vi "testTTL_v5.vi"() -> ()   [LabVIEW 2015]
uses:
  <vilib>/DAQmx/read.llb/DAQmx Read (Counter U32 1Chan 1Samp).vi
  <vilib>/DAQmx/write.llb/DAQmx Write (Analog Wfm 1Chan NSamp).vi
  <vilib>/DAQmx/write.llb/DAQmx Write (Digital Bool 1Line 1Point).vi
  <vilib>/DAQmx/create/channels.llb/DAQmx Create Channel (CI-Count Edges).vi
  <vilib>/DAQmx/miscellaneous.llb/DAQmx Fill In Error Info.vi
  <resource>/objmgr/daqmx.rc
panel:
  out "Phase offset (deg.)":dbl
  in  "Avg signal freq (Hz)":dbl
  out "level":sgl
  in  "Onboard counter":tag
  out "Counter error out":errorcluster
  in  "sample rate":dbl=30000.0
  in  "OEP sample clock in":tag="/Dev1/PFI1"
  in  "extra delay (samp)":i64
  out "Current OEP to LV delay (samp)":i64(graph)
  out "max delay (samp)":i64
  out "AO error out":errorcluster
  in  "Delay lock":bool
  out "DO error out":errorcluster
  out "time off (s)":dbl
  in  "Stop":bool
  out "time on (s)":dbl
  out "New event":bool
  in  "event channel":u8=1 min=1 max=8
  out "ZMQ error out":errorcluster
  in  "port":u16=5557
  # "*** Be sure to set analog and digital out channels in the PrepareChannels VI. ***"
  # "*** Start VI before starting OpenEphys acquisition for the sample count and delay measurements to be accurate. ***"
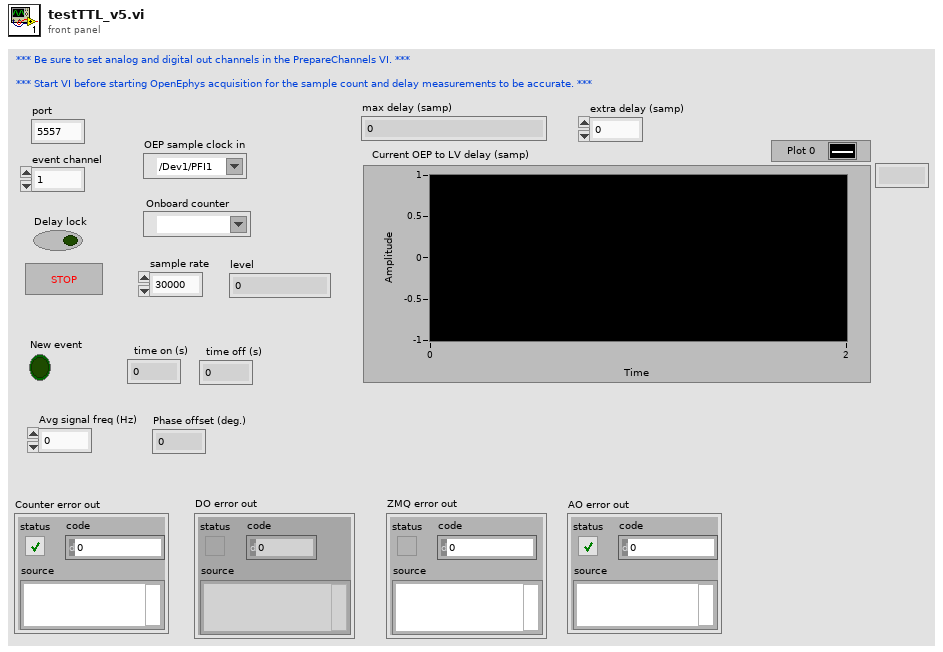
[diagram p1: front panel]
types:
  T1 = enum16{"big-endian, network order", "native, host order", "little-endian"}
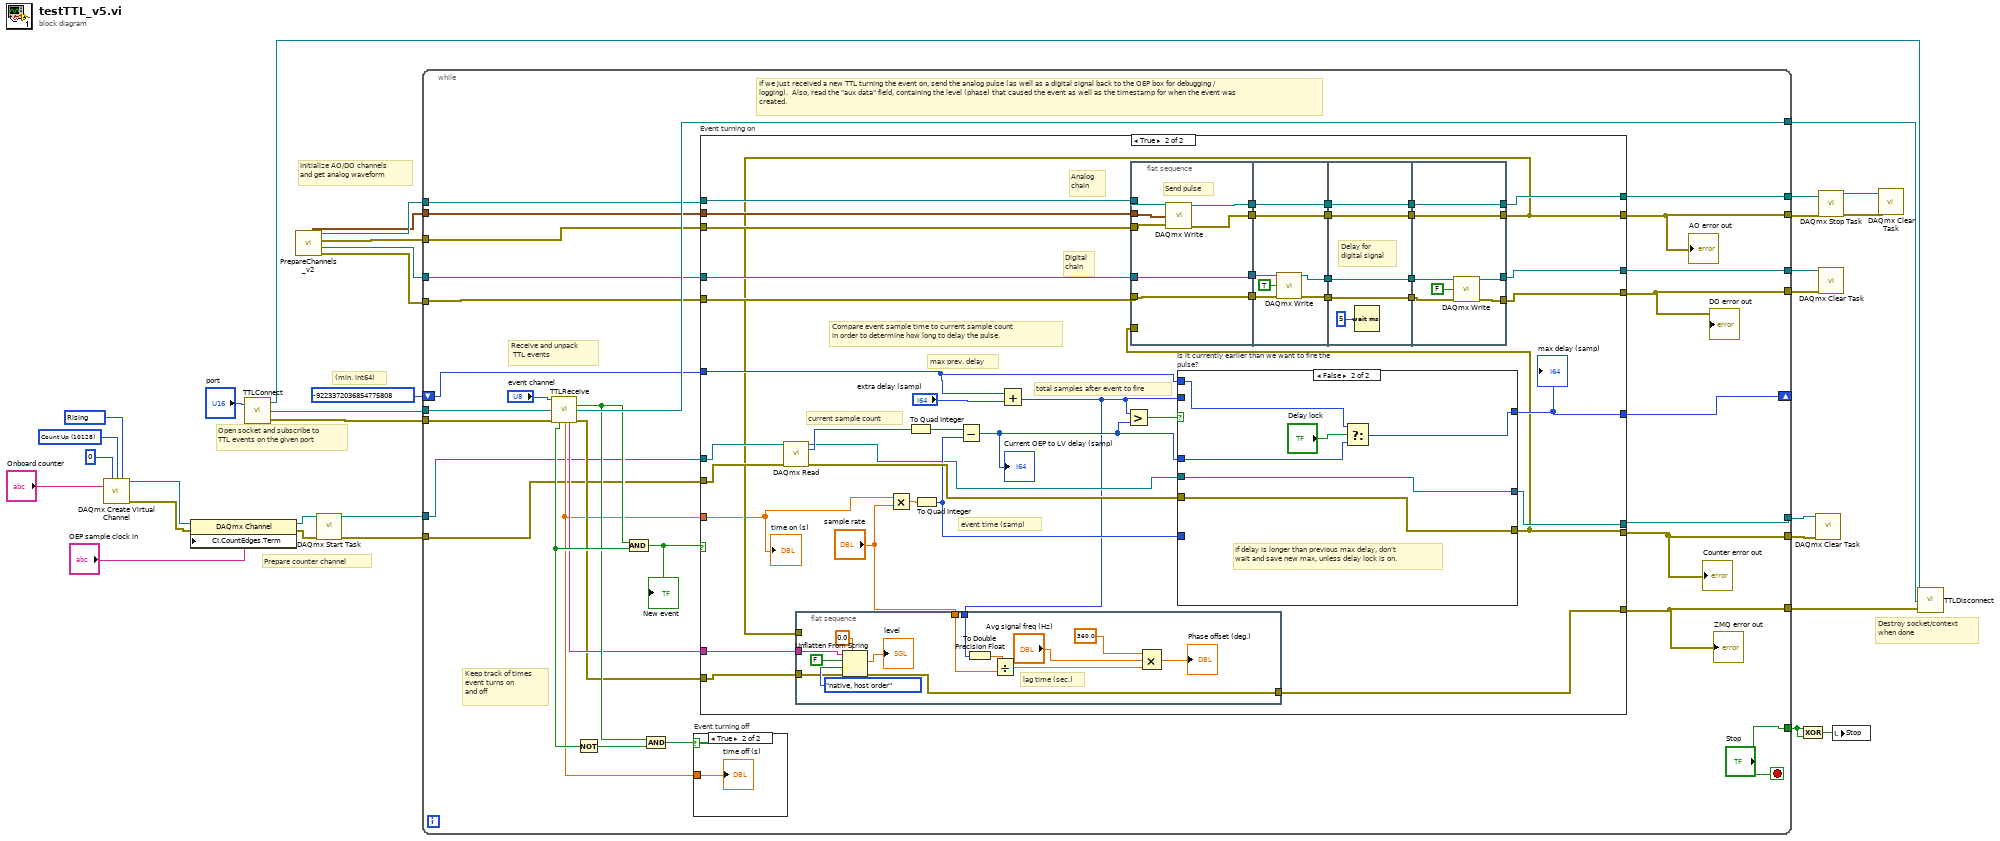
[diagram p0: block diagram]
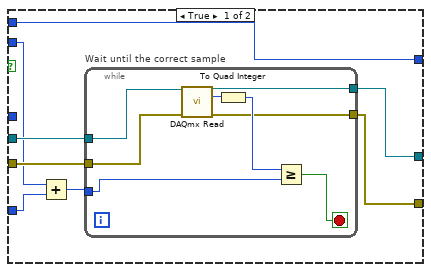
[diagram p3: hidden frame]
diagram:
  w10 = 10280 items=["Rising"=10280, "Falling"=10171] ("edge")
  w11 = 10128 items=["Count Up"=10128, "Count Down"=10124, "Externally Controlled"=10326] ("count direction")
  # "(min. int64)"
  # "Prepare counter channel"
  # "Initialize AO/DO channels\nand get analog waveform"
  # "Open socket and subscribe to\nTTL events on the given port"
  # "Destroy socket/context\nwhen done"
  n1 = call-poly <vilib>:"DAQmx Create Virtual Channel.vi"("initial count"=u32 0, "count direction"=w11, "edge"=w10, "counter"="Onboard counter") -> ("task out"=w14:refnum<k21>, "error out"=w13:errorcluster)  [unwired: 10 in]
  n2 = property class="DAQmx Channel"(reference=w14, error in=w13, "CI.CountEdges.Term"="OEP sample clock in") -> (reference out=w9:refnum<k21>, error out=w8:errorcluster)
  n3 = call "TTLConnect.vi"("port"="port") -> ("context out"=w32:refnum<class "zmq_context.lvclass">, "socket out"=w16:refnum<class "zmq_socket.lvclass">, "error out"=w17:errorcluster)  [unwired: 1 in]
  n4 = call "PrepareChannels_v2.vi"() -> ("DO error out"=w28:errorcluster, "DO task out"=w29:refnum<k21>, "AO error out"=w27:errorcluster, "AO task out"=w30:refnum<k21>, "Waveform Graph"=w22:waveform(dbl))  [unwired: 7 in]
  n5 = call <vilib>:"DAQmx Start Task.vi"("task/channels in"=w9, "error in"=w8) -> ("task out"=w7:refnum<k21>, "error out"=w6:errorcluster)  [unwired: 12 in]
  n6 = while {
    tunnel: w17 -> [w62]
    tunnel: [w39] -> w15
    tunnel: [w61] -> w31
    tunnel: w16 -> [w60]
    tunnel: w30 -> [w57]
    tunnel: w29 -> [w55]
    tunnel: w28 -> [w54]
    tunnel: w27 -> [w56]
    tunnel: [w44] -> w21
    tunnel: [w43] -> w20
    tunnel: [w47] -> w26
    tunnel: [w40] -> w25
    tunnel: ["Stop"] -> w24
    tunnel: w22 -> [w45]
    shift-right: [w41] -> _
    shift-left: i64 -9223372036854775808 -> [w42]
    tunnel: w7 -> [w37]
    tunnel: w6 -> [w36]
    tunnel: [w35] -> w5
    tunnel: [w34] -> w4
    stop <- "Stop" stop-if-true
    # "Receive and unpack\n TTL events"
    # "If we just received a new TTL turning the event on, send the analog pulse (as well as a digital signal back to the OEP box for debugging / logging).  Also, read the \"aux data\" field, containing the level (phase) that caused the event as well as the timestamp for when the event was created."
    # "Keep track of times\nevent turns on\nand off"
    n7 = call "TTLReceive.vi"("channel"="event channel", "socket in"=w60, "error in"=w62) -> ("new TTL"=w51:bool, "socket out"=w61:refnum<class "zmq_socket.lvclass">, "event on"=w52:bool, "timestamp (s)"=w38:dbl, "aux data"=w49:string, "error out"=w48:errorcluster)  [unwired: 6 in, 1 out]
    n8 = Not(x=w52) -> (.not. x?=w53:bool)
    n9 = And(x=w51, y=w52) -> (x .and. y?=w58:bool)
    "New event" <- w58
    n10 = And(x=w51, y=w53) -> (x .and. y?=w50:bool)
    n11 = case "Event turning off" shown="True" w50 {
      tunnel: w38 -> [_ w175]
      frame False {
      }
      frame True {
        "time off (s)" <- w175
      }
    }
    n12 = case "Event turning on" shown="True" w58 {
      tunnel: w57 -> [w70 w103]
      tunnel: w56 -> [w69 w100]
      tunnel: [w70 w101] -> w44
      tunnel: [w69 w75] -> w43
      tunnel: w55 -> [w67 w111]
      tunnel: w54 -> [w66 w105]
      tunnel: [w67 w112] -> w47
      tunnel: [w66 w108] -> w40
      tunnel: w38 -> [_ w72]
      tunnel: w49 -> [_ w77]
      tunnel: w48 -> [w68 w76]
      tunnel: [w68 w73] -> w39
      tunnel: w45 -> [_ w104]
      tunnel: w42 -> [w65 w99]
      tunnel: [w65 w106] -> w41
      tunnel: w37 -> [w64 w98]
      tunnel: w36 -> [w63 w90]
      tunnel: [w64 w88] -> w35
      tunnel: [w63 w81] -> w34
      frame False {
      }
      frame True {
        # "current sample count"
        # "total samples after event to fire"
        # "Compare event sample time to current sample count\nin order to determine how long to delay the pulse."
        # "event time (samp)"
        # "Digital\nchain"
        # "Analog \nchain"
        # "max prev. delay"
        n13 = call-poly <vilib>:"DAQmx Read.vi"("task/channels in"=w98, "error in"=w90) -> ("task out"=w89:refnum<k21>, "data"=w94:u32, "error out"=w92:errorcluster)  [unwired: 11 in]
        n14 = flat-sequence {
          tunnel: w77 -> [w122]
          tunnel: w76 -> [w121]
          tunnel: w75 -> [_]
          tunnel: w74 -> [w119]
          tunnel: [w120] -> w73
          tunnel: "sample rate" -> [w117]
          frame #0 {
            # "lag time (sec.)"
            n15 = Unflatten From String(type=sgl 0.0, binary string=w122, data includes array or string size? (T)=FALSE, byte order (0:big-endian, network order)=T1."native, host order", error in (no error)=w121) -> (value=→"level":sgl, error out=w120:errorcluster)  [unwired: 1 out]
            n16 = To Double Precision Float(number=w119) -> (double precision float=w118:dbl)
            n17 = Divide(x=w118, y=w117) -> (x/y=w116:dbl)
            n18 = Compound Arithmetic op=MULTIPLY(360.0 ("y"), "Avg signal freq (Hz)", w116) -> (→"Phase offset (deg.)":dbl)
          }
        }
        n19 = Multiply(x=w72, y="sample rate") -> (x*y=w96:dbl)
        n20 = To Quad Integer(1:w94) -> (0:w93:i64)
        n21 = To Quad Integer(1:w96) -> (0:w91:i64)
        n22 = Subtract(x=w93, y=w91) -> (x-y=w95:i64)
        "Current OEP to LV delay (samp)" <- w95
        n23 = Add(x=w99, y="extra delay (samp)") -> (x+y=w74:i64)
        n24 = Greater?(x=w74, y=w95) -> (0:w107:bool)
        n25 = flat-sequence {
          tunnel: [w155] -> w85
          tunnel: [w151] -> w83
          tunnel: [w150] -> w82
          tunnel: w105 -> [w150]
          tunnel: w111 -> [w151]
          tunnel: w100 -> [w153]
          tunnel: w104 -> [w154]
          tunnel: w103 -> [w152]
          tunnel: w81 -> [_]
          tunnel: [w149] -> w80
          tunnel: [w159] -> w87
          tunnel: [w157] -> w86
          tunnel: w85 -> [w162]
          tunnel: [w162] -> w84
          tunnel: w83 -> [w160]
          tunnel: w82 -> [w158]
          tunnel: w80 -> [w156]
          tunnel: [w156] -> w79
          tunnel: [w167] -> w110
          tunnel: w87 -> [w167]
          tunnel: [w166] -> w109
          tunnel: w86 -> [w166]
          tunnel: w84 -> [w164]
          tunnel: [w164] -> w102
          tunnel: w79 -> [w163]
          tunnel: [w163] -> w78
          tunnel: [w172] -> w112
          tunnel: w110 -> [w173]
          tunnel: w109 -> [w171]
          tunnel: [w170] -> w108
          tunnel: w102 -> [w169]
          tunnel: [w169] -> w101
          tunnel: [w168] -> w75
          tunnel: w78 -> [w168]
          frame #0 {
            # "Send pulse"
            n26 = call-poly <vilib>:"DAQmx Write.vi"("task/channels in"=w152, "data"=w154, "error in"=w153) -> ("task out"=w155:refnum<k21>, "error out"=w149:errorcluster)  [unwired: 10 in, 1 out]
          }
          frame #1 {
            n27 = call-poly <vilib>:"DAQmx Write.vi"("task/channels in"=w160, "data"=TRUE, "error in"=w158) -> ("task out"=w159:refnum<k21>, "error out"=w157:errorcluster)  [unwired: 10 in, 1 out]
          }
          frame #2 {
            # "Delay for \ndigital signal"
            n28 = Wait (ms)(milliseconds to wait=u32 5) -> ()  [unwired: 1 out]
          }
          frame #3 {
            n29 = call-poly <vilib>:"DAQmx Write.vi"("task/channels in"=w173, "data"=FALSE, "error in"=w171) -> ("task out"=w172:refnum<k21>, "error out"=w170:errorcluster)  [unwired: 10 in, 1 out]
          }
        }
        n30 = case "Is it currently earlier than we want to fire the pulse?" shown="False" w107 {
          tunnel: w95 -> [_ w144]
          tunnel: w99 -> [w134 w145]
          tunnel: [w134 w143] -> w106
          tunnel: w74 -> [w131 _]
          tunnel: w92 -> [w132 w148]
          tunnel: [w128 w148] -> w81
          tunnel: w91 -> [w130 _]
          tunnel: w89 -> [w133 w147]
          tunnel: [w127 w147] -> w88
          frame True {
            n31 = Add(x=w131, y=w130) -> (x+y=w129:i64)
            n32 = while "Wait until the correct sample" {
              tunnel: w133 -> [w141]
              tunnel: w132 -> [w142]
              tunnel: w129 -> [w140]
              tunnel: [w136] -> w128
              tunnel: [w135] -> w127
              stop <- w139 stop-if-true
              n33 = call-poly <vilib>:"DAQmx Read.vi"("task/channels in"=w141, "error in"=w142) -> ("task out"=w135:refnum<k21>, "data"=w138:u32, "error out"=w136:errorcluster)  [unwired: 11 in]
              n34 = To Quad Integer(1:w138) -> (0:w137:i64)
              n35 = Greater Or Equal?(x=w137, y=w140) -> (x >= y?=w139:bool)
            }
          }
          frame False, Default {
            # "If delay is longer than previous max delay, don't\nwait and save new max, unless delay lock is on."
            n36 = Select(t=w145, s="Delay lock", f=w144) -> (s? t:f=w143:i64)
          }
        }
        "max delay (samp)" <- w106
        "time on (s)" <- w72
      }
    }
    "DO error out" <- w40
    "AO error out" <- w43
    "ZMQ error out" <- w39
    "Counter error out" <- w34
  }
  n37 = Exclusive Or(1:w24, 2:w24) -> (0:w23:bool)
  n38 = call <vilib>:"DAQmx Clear Task.vi"("task in"=w5, "error in"=w4) -> ()  [unwired: 13 in, 1 out]
  n39 = call <vilib>:"DAQmx Stop Task.vi"("task/channels in"=w21, "error in"=w20) -> ("task out"=w19:refnum<k21>, "error out"=w18:errorcluster)  [unwired: 12 in]
  n40 = call <vilib>:"DAQmx Clear Task.vi"("task in"=w26, "error in"=w25) -> ()  [unwired: 13 in, 1 out]
  n41 = local write "Stop"(w23) -> ()
  n42 = call <vilib>:"DAQmx Clear Task.vi"("task in"=w19, "error in"=w18) -> ()  [unwired: 13 in, 1 out]
  n43 = call "TTLDisconnect.vi"("error in"=w15, "socket in"=w31, "context in"=w32) -> ()  [unwired: 1 in, 1 out]
